vi "Time Filter Data (LV Dbl).vi"(4 "End":dbl, 6 "Start":dbl, 10 "Group Data":T2) -> (2 "Data":T1[](array[typedef]))   [LabVIEW 2020, in "VolatusHistorian.lvlib" / "Historian Module.lvclass"]
uses:
  Group Data.ctl
  Channel Data.ctl
  lv-vecto/Vecto/Double to Relative ns (Array).vi
  Historian Module.lvclass
  Historian Module.lvclass/Historian Module.ctl
  Channel History (LV Dbl).ctl
  VolatusHistorian.lvlib
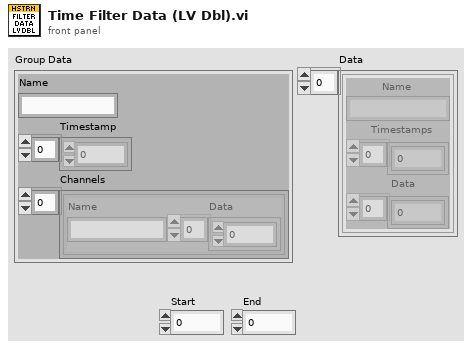
[diagram p1: front panel]
types:
  T1 = typedef "VolatusHistorian.lvlib/Channel History (LV Dbl).ctl" = cluster{"Name":string, "Timestamps":dbl[], "Data":dbl[]}
  T2 = typedef "VolatusHistorian.lvlib/Group Data.ctl" = cluster{"Name":string, "Timestamp":dbl[], "Channels":T3[]}
  T3 = typedef "VolatusHistorian.lvlib/Channel Data.ctl" = cluster{"Name":string, "Data":dbl[]}
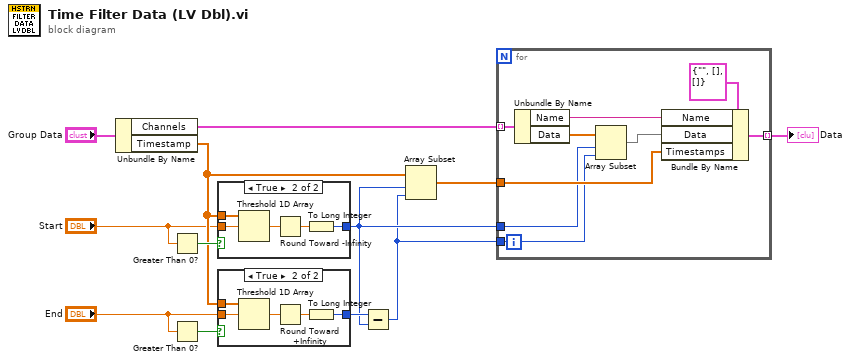
[diagram p0: block diagram]
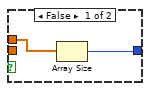
[diagram p2: hidden frame]
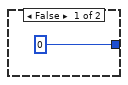
[diagram p3: hidden frame]
diagram:
  n1 = Unbundle By Name("Group Data") -> ("Channels"=w8:T3[], "Timestamp"=w9:dbl[])
  n2 = Greater Than 0?(x="Start") -> (x > 0?=w12:bool)
  n3 = Greater Than 0?(x="End") -> (x > 0?=w11:bool)
  n4 = case shown="True" w12 {
    tunnel: w9 -> [_ w16]
    tunnel: "Start" -> [_ w18]
    tunnel: [0 w15] -> w7
    frame False {
    }
    frame True {
      n5 = Threshold 1D Array(2:w18, 3:w16) -> (0:w17:dbl)  [unwired: 1 in]
      n6 = Round Toward -Infinity(1:w17) -> (0:w14:dbl)
      n7 = To Long Integer(number=w14) -> (32bit integer=w15:i32)
    }
  }
  n8 = case shown="True" w11 {
    tunnel: w9 -> [w20 w23]
    tunnel: "End" -> [_ w25]
    tunnel: [w19 w22] -> w10
    frame False {
      n9 = Array Size(array=w20) -> (size(s)=w19:i32)
    }
    frame True {
      n10 = Threshold 1D Array(2:w25, 3:w23) -> (0:w24:dbl)  [unwired: 1 in]
      n11 = Round Toward +Infinity(x=w24) -> (ceil(x): smallest int >= x=w21:dbl)
      n12 = To Long Integer(number=w21) -> (32bit integer=w22:i32)
    }
  }
  n13 = Subtract(x=w10, y=w7) -> (x-y=w6:i32)
  n14 = Array Subset(array=w9, index=w7, length=w6) -> (w1:dbl[])
  n15 = for {
    tunnel: w8 -> [w32] mode=indexing
    tunnel: w1 -> [w33]
    tunnel: w7 -> [w29]
    tunnel: w6 -> [w27]
    tunnel: [w26] -> w5 mode=indexing
    n16 = Unbundle By Name(w32) -> ("Name"=w31:string, "Data"=w30:dbl[])
    n17 = Array Subset(array=w30, index=w29, length=w27) -> (w28:dbl[])
    n18 = Bundle By Name(cluster=T1 {"Name"="", "Timestamps"=[], "Data"=[]} ("Local Channel"), "Name"=w31, "Data"=w28, "Timestamps"=w33) -> (w26:T1)
  }
  "Data" <- w5
